vi "wait for plc bit and abort.vi"(8 "error in":errorcluster, 9 "tag":T2 {"DataSocket Reference"."OnStatusUpdated" format="%.0x"; "DataSocket Reference"."OnDataUpdated" format="%.0x"}, 11 "Abort Test":T1) -> (0 "error out":errorcluster, 2 "final values":bool)   [LabVIEW 2018]
uses:
  05.UserVI's/type defs/plc path and tag.ctl
  <vilib>/Platform/dataskt.llb/DataSocket Reference Type.ctl
  05.UserVI's/type defs/EOL Global Digital Input Control.ctl
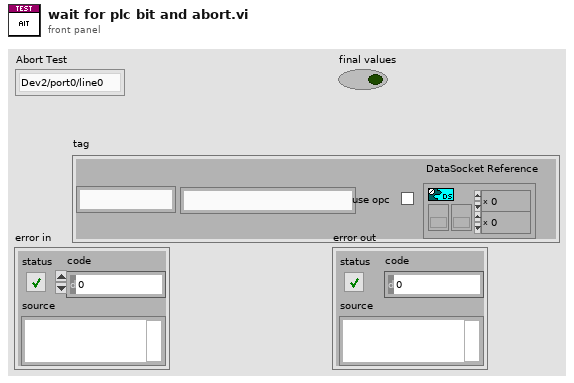
[diagram p1: front panel]
types:
  T1 = typedef "EOL Global Digital Input Control.ctl" = enum16{"Dev2/port0/line0", "Dev2/port0/line1", "Dev2/port0/line2", "Dev2/port0/line3", "Dev2/port0/line4", "Dev2/port0/line5", "Dev2/port0/line6", "Dev2/port0/line7", "Dev2/port1/line0", "Dev2/port1/line1", "Dev2/port1/line2", "Dev2/port1/line3", "Dev2/port1/line4", "Dev2/port1/line5", "Dev2/port1/line6", "Dev2/port1/line7", "Dev2/port2/line0", "Dev2/port2/line1", "Dev2/port2/line2", "Dev2/port2/line3", "Dev2/port2/line4", "Dev2/port2/line5", "Dev2/port2/line6", "Dev2/port2/line7", "Prerun Start Test", "Prerun Abort Test", "Audit Start Test", "Audit Abort Test", "Dev2/port3/line4", "Dev2/port3/line5", "Breakin Start Test", "Breakin Abort Test", "Not Implemented"}
  T2 = typedef "plc path and tag.ctl" = cluster{"Tag Name":string, "Network Path":string, "use opc":bool, "DataSocket Reference":T3}
  T3 = typedef "DataSocket Reference Type.ctl" = cluster{"CWDSLib._DCWDataSocket":refnum<k7>, "CWDSLib._DCWData":refnum<k7>, "OnDataUpdated":u32, "OnStatusUpdated":u32}
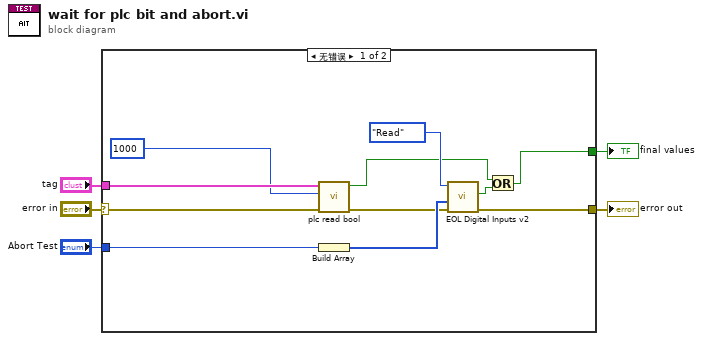
[diagram p0: block diagram]
diagram:
  n1 = case shown="无错误" "error in" {
    selector: "error in" -> [w12 w17]
    tunnel: "tag" -> [w16 _]
    tunnel: "Abort Test" -> [w15 _]
    tunnel: [w14 w17] -> w3
    tunnel: [w6 _] -> w2
    frame No Error {
      n2 = call "plc read bool.vi"("error in"=w12, "Timeout (ms)"=1000 ("milliseconds to wait"), "addr,tag"=w16) -> ("error out"=w9:errorcluster, "value"=w7:bool)  [unwired: 7 in]
      n3 = Build Array(w15) -> (w10:T1[])
      n4 = call "EOL Digital Inputs v2.vi"("Sys Error In"=w9, "Digital Inputs Array"=w10, "Mode"=enum16{"Init", "Read", "Read All", "Close"}."Read") -> ("Sys Error Out"=w14:errorcluster, "Single Input"=w8:bool)  [unwired: 6 in, 1 out]
      n5 = Or(x=w7, y=w8) -> (x .or. y?=w6:bool)
    }
    frame Error {
    }
  }
  "error out" <- w3
  "final values" <- w2
